vi "test_Mono_Setup_Testenvironment.vi"(8 "error in":errorcluster) -> (0 "error out":errorcluster, 2 "device open for communication?":bool, 3 "Monochromator out":refnum<class "Monochromator.lvclass">)   [LabVIEW 2023]
uses:
  Classes/Mono/Monochromator.lvclass
  Libraries/DeviceManager/DeviceManager.lvlib
panel:
  # "Connector Pane"
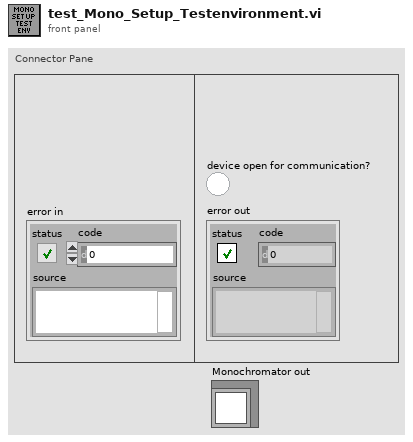
[diagram p1: front panel]
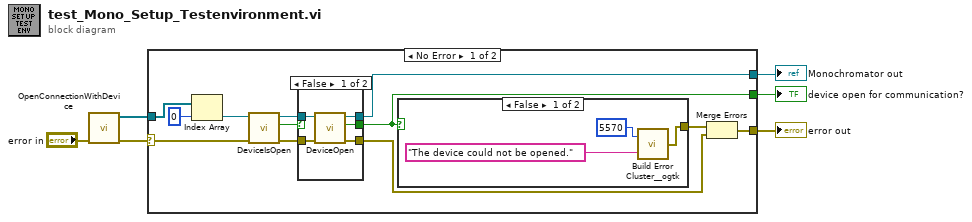
[diagram p0: block diagram]
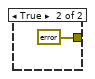
[diagram p3: hidden frame]
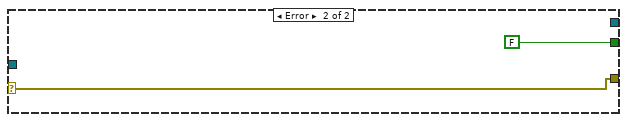
[diagram p4: hidden frame]
diagram:
  n1 = call "OpenConnectionWithDevice.vi"("error in"="error in") -> ("error out"=w2:errorcluster, "Monos"=w1:refnum<class "Monochromator.lvclass">[])  [unwired: 7 in, 2 out]
  n2 = case shown="No Error" w2 {
    selector: w2 -> [w10 w32]
    tunnel: w1 -> [w18 _]
    tunnel: [w16 w32] -> w5
    tunnel: [w14 FALSE ("CCD open for communication?")] -> w4
    tunnel: [w12 _] -> w3
    frame No Error {
      n3 = Index Array(array=w18, index=0) -> (element=w11:refnum<class "Monochromator.lvclass">)
      n4 = call-dynamic "DeviceIsOpen.vi"("error in (no error)"=w10, "Monochromator in"=w11) -> ("error out"=w9:errorcluster, "device is open?"=w8:bool, "Monochromator out"=w7:refnum<class "Monochromator.lvclass">)  [unwired: 6 in, 1 out]
      n5 = case shown="False" w8 {
        selector: w8 -> [_ w24]
        tunnel: [w23 w24] -> w14
        tunnel: [w22 w25] -> w13
        tunnel: [w21 w26] -> w12
        tunnel: w9 -> [w20 w25]
        tunnel: w7 -> [w19 w26]
        frame False {
          n6 = call-dynamic "DeviceOpen.vi"("error in (no error)"=w20, "Monochromator in"=w19) -> ("error out"=w22:errorcluster, "device is open?"=w23:bool, "Monochromator out"=w21:refnum<class "Monochromator.lvclass">)  [unwired: 6 in, 1 out]
        }
        frame True {
        }
      }
      n7 = case shown="False" w14 {
        tunnel: [w28 errorcluster {"status"=FALSE, "code"=0, "source"=""} ("error in 2")] -> w15
        frame False {
          n8 = call <userlib>:"Build Error Cluster__ogtk.vi"("String to Prepend to source (\"\")"="The device could not be opened." ("String to Prepend to source (\"\")"), "code"=5570) -> ("error out"=w28:errorcluster)
        }
        frame True {
        }
      }
      n9 = Merge Errors(w15, w13) -> (w16:errorcluster)
    }
    frame Error {
    }
  }
  "error out" <- w5
  "device open for communication?" <- w4
  "Monochromator out" <- w3
